vi "VISA response check.vi"(0 "Cobolt in":refnum<class "Cobolt.lvclass">, 11 "error in (no error)":errorcluster) -> (4 "Cobolt out":refnum<class "Cobolt.lvclass">, 6 "ResponseOK":bool, 10 "Retry":bool, 15 "error out":errorcluster)   [LabVIEW 2012, in "Cobolt.lvclass"]
uses:
  Cobolt.lvclass
  Cobolt.lvclass/Cobolt.ctl
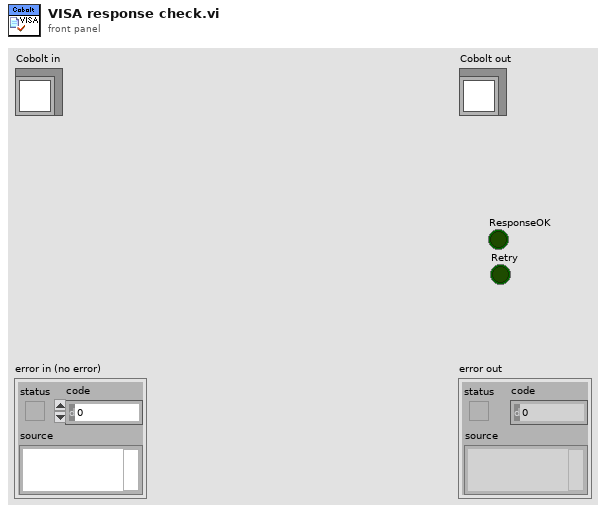
[diagram p1: front panel]
types:
  T1 = typedef "Cobolt.lvclass/ExpectedResponseType.ctl" = u16
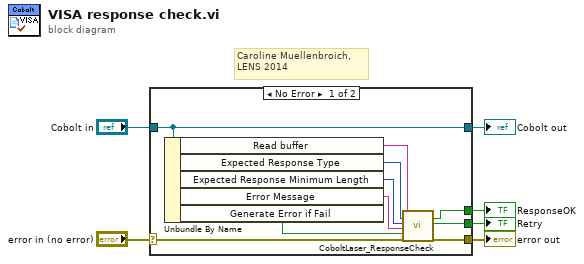
[diagram p0: block diagram]
diagram:
  # "Caroline Muellenbroich, \nLENS 2014"
  n1 = case shown="No Error" "error in (no error)" {
    selector: "error in (no error)" -> [w16 w18]
    tunnel: [w15 w18] -> w5
    tunnel: [w12 w17] -> w3
    tunnel: "Cobolt in" -> [w12 w17]
    tunnel: [w14 _] -> w2
    tunnel: [w13 _] -> w1
    frame No Error {
      n2 = Unbundle By Name(w12) -> ("Read buffer"=w11:string, "Expected Response Type"=w10:T1, "Expected Response Minimum Length"=w9:i32, "Error Message"=w8:string, "Generate Error if Fail"=w7:bool)
      n3 = call "CoboltLaser_ResponseCheck.vi"("Response"=w11, "ExpectedResponseType"=w10, "ExpectedResponseMinimumLength"=w9, "ErrorMessage"=w8, "GenerateErrorIfFail"=w7, "ErrorIn"=w16) -> ("ResponseOK"=w14:bool, "Retry"=w13:bool, "ErrorOut"=w15:errorcluster)  [unwired: 11 in]
    }
    frame Error {
    }
  }
  "error out" <- w5
  "Cobolt out" <- w3
  "ResponseOK" <- w2
  "Retry" <- w1
